vi "Marshal.vi"(8 "error in (no error)":errorcluster, 11 "Type Serializer in":refnum<class "Type Serializer.lvclass">) -> (0 "error out":errorcluster, 2 "Buffer":u8[](array[numeric]), 3 "Type Serializer out":refnum<class "Type Serializer.lvclass">)   [LabVIEW 2020, in "Protobuf RAW.lvlib" / "Type Serializer.lvclass"]
uses:
  Type Serializer.lvclass
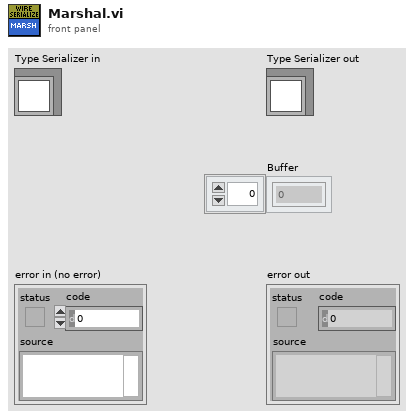
[diagram p1: front panel]
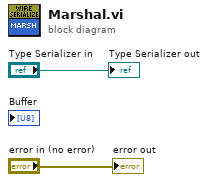
[diagram p0: block diagram]
diagram:
  "error out" <- "error in (no error)"
  "Type Serializer out" <- "Type Serializer in"
